vi "WristAtSetpoint.vi"() -> (3 "WristAtSetpoint":bool)   [LabVIEW 2023]
doc: "Checks if actual Wrist position is within 1 degree of setpoint"
uses:
  WristGlobal.vi
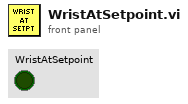
[diagram p1: front panel]
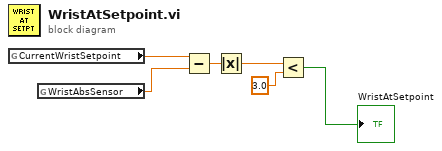
[diagram p0: block diagram]
diagram:
  n1 = global read "WristGlobal.vi" "CurrentWristSetpoint"() -> (w6:dbl)
  n2 = global read "WristGlobal.vi" "WristAbsSensor"() -> (w5:dbl)
  n3 = Subtract(x=w6, y=w5) -> (x-y=w4:dbl)
  n4 = Absolute Value(x=w4) -> (abs(x)=w3:dbl)
  n5 = Less?(x=w3, y=3.0) -> (x < y?=→"WristAtSetpoint":bool)
